vi "onTheFlyCal.vi"(8 "error in (no error)":errorcluster, 10 "calibrateElevator":bool, 11 "Elevator Linear in":refnum<class "Elevator Linear.lvclass">) -> (0 "error out":errorcluster, 3 "Elevator Linear out":refnum<class "Elevator Linear.lvclass">)   [LabVIEW 2019, in "Elevator.lvlib" / "Elevator Linear.lvclass"]
doc: "Calibrates the elevator by making go downwards until it hits a limit switch if it wasnt on the limit switch in begin or you press a button"
uses:
  Elevator Linear.lvclass
  C:/Users/Public/Documents/2020InfinteRecharge/src robot/Classes/Elevator/Elevator.lvclass
  Elevator Linear.lvclass/Elevator Linear.ctl
  <vilib>/Rock Robotics/WPI/ThirdParty/Phoenix-LabVIEW/Motor Controller/Controls/CTRE_Phoenix_MotorControl_ControlMode.ctl
  <vilib>/Rock Robotics/WPI/ThirdParty/Phoenix-LabVIEW/Motor Controller/Get/CTRE_Phoenix_MotorController_GetLimitSwitchStates.vi
  Elevator.lvclass
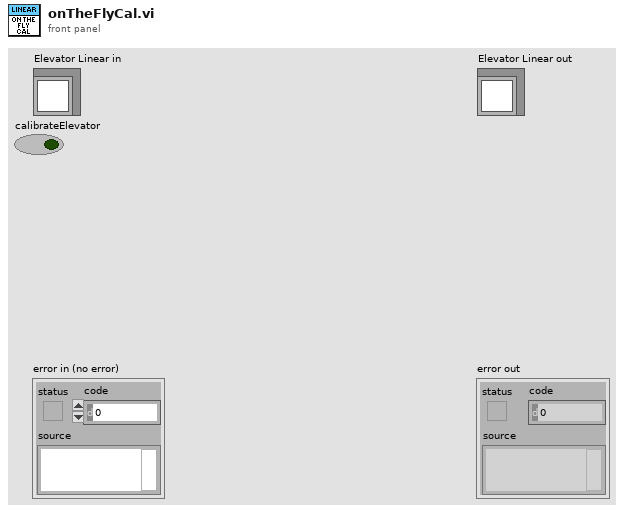
[diagram p1: front panel]
types:
  T1 = typedef "Elevator.lvlib/Elevator.lvclass/Elevator Constants.ctl" = cluster{"Arm Motion Magic Max Velocity":u32, "Arm Motion Magic Max Acceleration":u32, "Wrist Motion Magic Max Velocity":u32, "Wrist Motion Magic Max Acceleration":u32, "Elevator Linear Motion Magic Max Velocity":u32, "Elevator Linear Motion Magic Max Acceleration":u32, "Arm Gear Ratio":dbl, "Wrist Gear Ratio":dbl, "Elevator Linear Gear Ratio":dbl, "Arm Encoder ABS Value":i32, "Wrist Encoder ABS Value":i32}
  T2 = typedef "CTRE_Phoenix_MotorControl_ControlMode.ctl" = u16
  T3 = typedef "WPI_MotorControlDeviceRef.ctl" = cluster{"DeviceStatus":errorcluster, "Type":T4, "PWM":cluster{"PWM Channel":T5, "DeadBand":T6}, "CAN":cluster{"Device Number":u8, "SetOutput VI Ref":variant, "GetOutput VI Ref":variant, "Enable VI Ref":variant, "Disable VI Ref":variant, "Data":variant}, "Invert":bool, "DIO PWM":cluster{"PWM \"Enable\" Channel":T5, "DIOChannel":T7, "PWM Rate":dbl}}
  T4 = typedef "WPI_MotorControlType.ctl" = enum16{"PWM", "CAN", "DIO PWM"}
  T5 = typedef "FPGA_DIOPWMChannel.ctl" = enum8{"PWM 0", "PWM 1", "PWM 2", "PWM 3", "PWM 4", "PWM 5", "PWM 6", "PWM 7", "PWM 8", "PWM 9", "PWM MXP 0", "PWM MXP 1", "PWM MXP 2", "PWM MXP 3", "PWM MXP 4", "PWM MXP 5", "PWM MXP 6", "PWM MXP 7", "PWM MXP 8", "PWM MXP 9", "Invalid"}
  T6 = typedef "WPI_PWMDeadband.ctl" = cluster{"Name":string, "maxPositivePwm":i32, "minPositivePwm":i32, "centerPwm":i32, "maxNegativePwm":i32, "minNegativePwm":i32, "angularRange":u16}
  T7 = typedef "FPGA_DIOChannel.ctl" = enum8{"DIO 0", "DIO 1", "DIO 2", "DIO 3", "DIO 4", "DIO 5", "DIO 6", "DIO 7", "DIO 8", "DIO 9", "DIO MXP 0", "DIO MXP 1", "DIO MXP 2", "DIO MXP 3", "DIO MXP 4", "DIO MXP 5", "DIO MXP 6", "DIO MXP 7", "DIO MXP 8", "DIO MXP 9", "DIO MXP 10", "DIO MXP 11", "DIO MXP 12", "DIO MXP 13", "DIO MXP 14", "DIO MXP 15", "SPI Port CS1", "SPI Port CS2", "SPI Port CS3", "SPI Port MISO", "SPI Port MOSI", "Invalid"}
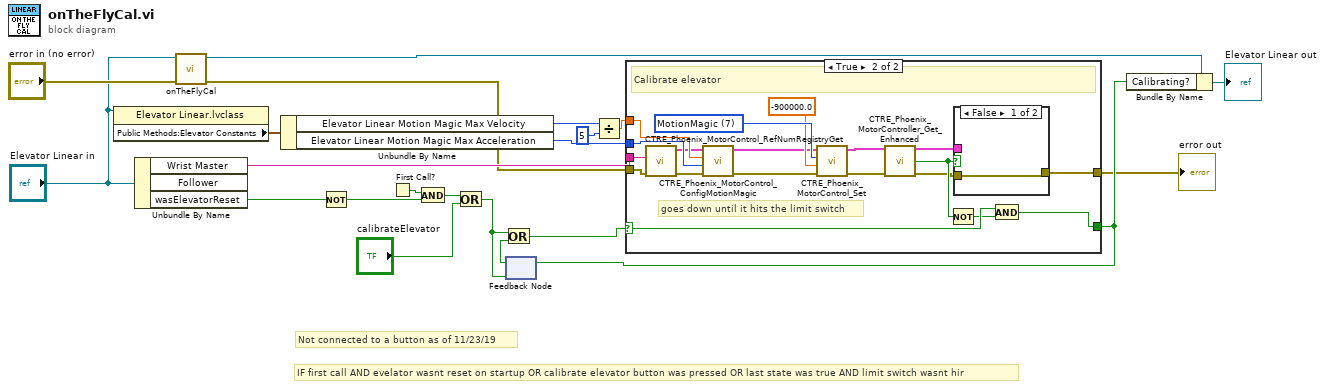
[diagram p0: block diagram]
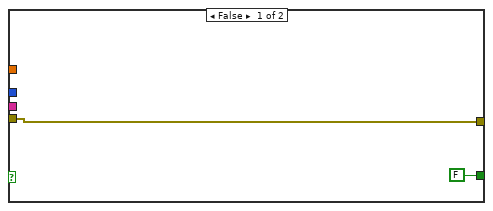
[diagram p2: hidden frame]
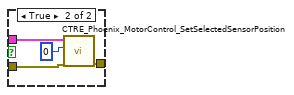
[diagram p3: hidden frame]
diagram:
  # "Not connected to a button as of 11/23/19"
  # "IF first call AND evelator wasnt reset on startup OR calibrate elevator button was pressed OR last state was true AND limit switch wasnt hir"
  n1 = property class="Elevator Linear.lvclass"(reference="Elevator Linear in") -> ("Public Methods:Elevator Constants"=w7:T1)  [unwired: 1 in, 2 out]
  n2 = Unbundle By Name("Elevator Linear in") -> ("Wrist Master"=w19:string, "wasElevatorReset"=w20:bool)  [unwired: 1 out]
  n3 = call-parent "onTheFlyCal.vi"("error in (no error)"="error in (no error)", "Elevator in"="Elevator Linear in") -> ("error out"=w2:errorcluster, "Elevator out"=w11:refnum<class "Elevator Linear.lvclass">)  [unwired: 8 in]
  n4 = Unbundle By Name(w7) -> ("Elevator Linear Motion Magic Max Velocity"=w6:u32, "Elevator Linear Motion Magic Max Acceleration"=w4:u32)
  n5 = Not(x=w20) -> (.not. x?=w12:bool)
  n6 = First Call?() -> (First Call?: T/F=w13:bool)
  n7 = And(x=w13, y=w12) -> (x .and. y?=w18:bool)
  n8 = Or(x=w18, y="calibrateElevator") -> (x .or. y?=w14:bool)
  n9 = feedback #1(w14) -> (w15:bool)
  n10 = Or(x=w14, y=w15) -> (x .or. y?=w16:bool)
  n11 = Divide(x=w6, y=u32 5) -> (x/y=w3:dbl)
  n12 = case shown="True" w16 {
    selector: w16 -> [_ w37]
    tunnel: w19 -> [_ w42]
    tunnel: [FALSE w36] -> w10
    tunnel: w4 -> [_ w32]
    tunnel: w3 -> [_ w31]
    tunnel: w2 -> [w22 w26]
    tunnel: [w22 w24] -> w1
    frame False {
    }
    frame True {
      w41 = T2 7 items=["PercentOutput"=0, "Position"=1, "Velocity"=2, "Current"=3, "Follower"=5, "MotionProfile"=6, "MotionMagic"=7, "MotionProfileArc"=10, "Disabled"=15] ("Control Mode")
      # "goes down until it hits the limit switch"
      # "Calibrate elevator"
      n13 = call <vilib>:"CTRE_Phoenix_MotorControl_RefNumRegistryGet.vi"("error in (no error)"=w26, "refnum name"=w42) -> ("error out"=w29:errorcluster, "PhoenixMotorControlDevRef"=w30:T3)  [unwired: 8 in]
      n14 = call <vilib>:"CTRE_Phoenix_MotorControl_ConfigMotionMagic.vi"("error in (no error)"=w29, "Acceleration"=w32, "Cruise Velocity"=w31, "PhoenixMotorControlDevRef"=w30) -> ("error out"=w28:errorcluster, "PhoenixMotorControlDevRef"=w27:T3)  [unwired: 6 in]
      n15 = call <vilib>:"CTRE_Phoenix_MotorControl_Set.vi"("error in (no error)"=w28, "Output"=-900000.0, "Control Mode"=w41, "PhoenixMotorControlDevRef"=w27) -> ("error out"=w38:errorcluster, "PhoenixMotorControlDevRef"=w39:T3)  [unwired: 6 in]
      n16 = call-poly <vilib>:"CTRE_Phoenix_MotorController_Get_Enhanced.vi"("PhoenixMotorControlDevRef"=w39, "error in"=w38) -> ("PhoenixMotorControlDevRef"=w33:T3, "Reverse Limit Closed?"=w34:bool, "error out"=w25:errorcluster)  [unwired: 10 in, 1 out]
      n17 = Not(x=w34) -> (.not. x?=w35:bool)
      n18 = case shown="False" w34 {
        tunnel: w33 -> [_ w47]
        tunnel: w25 -> [w43 w45]
        tunnel: [w43 w44] -> w24
        frame False {
        }
        frame True {
          n19 = call <vilib>:"CTRE_Phoenix_MotorControl_SetSelectedSensorPosition.vi"("error in (no error)"=w45, "New Sensor Position"=0, "PhoenixMotorControlDevRef"=w47) -> ("error out"=w44:errorcluster)  [unwired: 7 in, 1 out]
        }
      }
      n20 = And(x=w37, y=w35) -> (x .and. y?=w36:bool)
    }
  }
  "error out" <- w1
  n21 = feedback-in #1(w10) -> ()
  n22 = Bundle By Name(cluster=w11, "Calibrating?"=w10) -> (→"Elevator Linear out":refnum<class "Elevator Linear.lvclass">)
